vi "move to next scan.vi"(6 "Step size":dbl, 8 "Speed":i32, 9 "Scan index":i32, 10 "error in (no error)":errorcluster, 11 "CNC COM in":refnum<visa-resource-name>) -> (0 "error out":errorcluster, 3 "CNC COM out":refnum<visa-resource-name>)   [LabVIEW 2014]
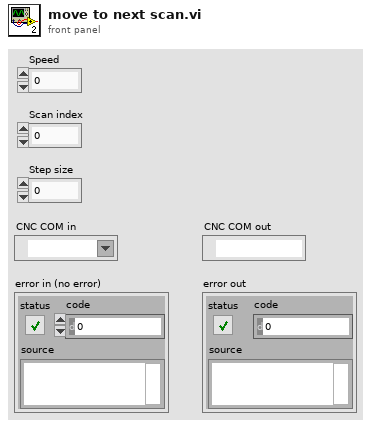
[diagram p1: front panel]
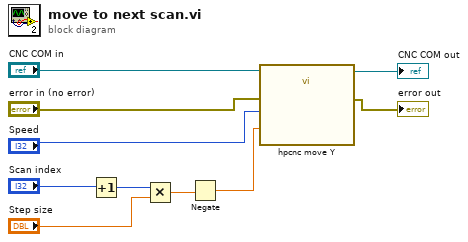
[diagram p0: block diagram]
diagram:
  n1 = Increment(x="Scan index") -> (x+1=w2:i32)
  n2 = Multiply(x=w2, y="Step size") -> (x*y=w1:dbl)
  n3 = Negate(x=w1) -> (-x=w5:dbl)
  n4 = call "hpcnc move Y.vi"("VISA Refnum in"="CNC COM in", "Y"=w5, "Speed"="Speed", "error in"="error in (no error)") -> ("VISA Refnum out"=→"CNC COM out":refnum<visa-resource-name>, "error out"=→"error out":errorcluster)  [unwired: 14 in]
